vi "JudgeXZ.vi"(8 "错误输入":errorcluster caption="StepError", 10 "Z Right Limit":bool, 11 "com in":refnum<visa-resource-name>) -> (0 "错误输出":errorcluster caption="StepError", 3 "com out":refnum<visa-resource-name>)   [LabVIEW 2018]
uses:
  Device VIs/Verbal.vi
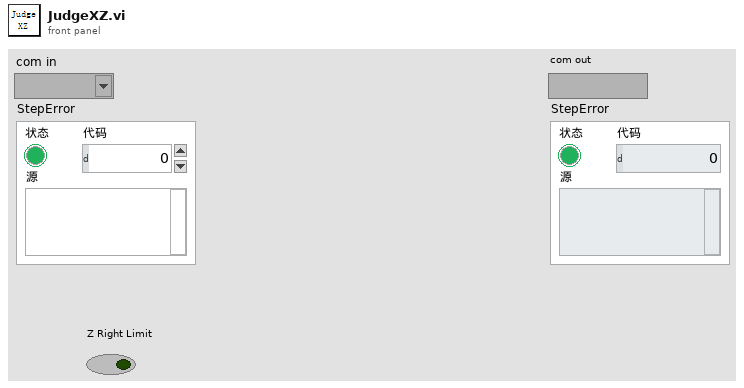
[diagram p1: front panel]
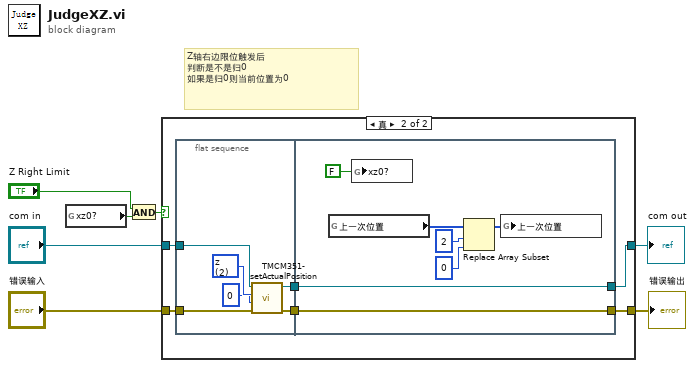
[diagram p0: block diagram]
diagram:
  # "Z轴右边限位触发后\n判断是不是归0\n如果是归0则当前位置为0"
  n1 = global read "Verbal.vi" "xz0?"() -> (w4:bool)
  n2 = And(x="Z Right Limit", y=w4) -> (x .and. y?=w3:bool)
  n3 = case shown="真" w3 {
    tunnel: "错误输入" -> [w8 w15]
    tunnel: "com in" -> [w9 w14]
    tunnel: [w9 w13] -> w2
    tunnel: [w8 w12] -> w1
    frame False {
    }
    frame True {
      n4 = flat-sequence {
        tunnel: w15 -> [w21]
        tunnel: w14 -> [w20]
        tunnel: [w17] -> w11
        tunnel: [w16] -> w10
        tunnel: [w27] -> w12
        tunnel: [w28] -> w13
        tunnel: w11 -> [w28]
        tunnel: w10 -> [w27]
        frame #0 {
          w19 = u8 2 items=["x", "y", "z"] ("motor")
          n5 = call "TMCM351- setActualPosition.vi"("错误输入"=w21, "Position"=0, "motor"=w19, "com in"=w20) -> ("错误输出"=w16:errorcluster, "com out"=w17:refnum<visa-resource-name>)  [unwired: 2 in]
        }
        frame #1 {
          n6 = global read "Verbal.vi" "上一次位置"() -> (w25:i32[])
          n7 = global write "Verbal.vi" "xz0?"(FALSE ("xz0?")) -> ()
          n8 = Replace Array Subset(array=w25, new element=0 ("新元素/子数组"), index=2 ("索引")) -> (w22:i32[])
          n9 = global write "Verbal.vi" "上一次位置"(w22) -> ()
        }
      }
    }
  }
  "com out" <- w2
  "错误输出" <- w1
